vi "CRYView Model CurLibrary.vi"(8 "sOption":string, 9 "nData":i32, 10 "sData":string, 11 "sAction":string) -> (0 "bResult":bool=TRUE, 1 "pRefList_Out":variant[](array[variant]), 2 "pVIRef_Out":refnum<vi>, 3 "SData_Out":string)   [LabVIEW 2013]
uses:
  CRYNew View Global.vi
  CRYView Global.vi
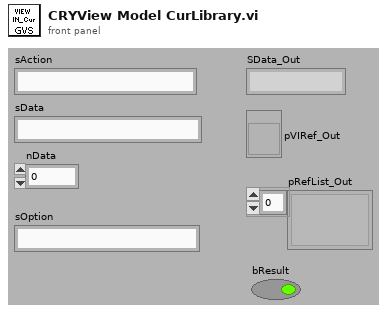
[diagram p1: front panel]
types:
  T1 = typedef "Graph Main Info Cluster.ctl" = cluster{"Selected_BarIdx":i32, "Selected_PanelIdx":i32, "Graph Main VIRef":refnum<vi>, "ToolBarClick":bool, "Spliter Ref Array":refnum<vi>[], "Panel Ref Array":refnum<vi>[], "Spliter_matrix":i32[][], "Panel_matrix":i32[][], "child_spliterIdx_matrix":i32[][], "split_pos_matrix":i32[][], "Title State":bool, "sQueueName":string, "Frame nID":i32, "Graph VIRef Array":cluster{"Graph VIRef":refnum<vi>, "Panel Idx":i32, "Frame VIRef":refnum<vi>, "Icon Ring":i32, "Graph Type":string}[], "View Type":string}
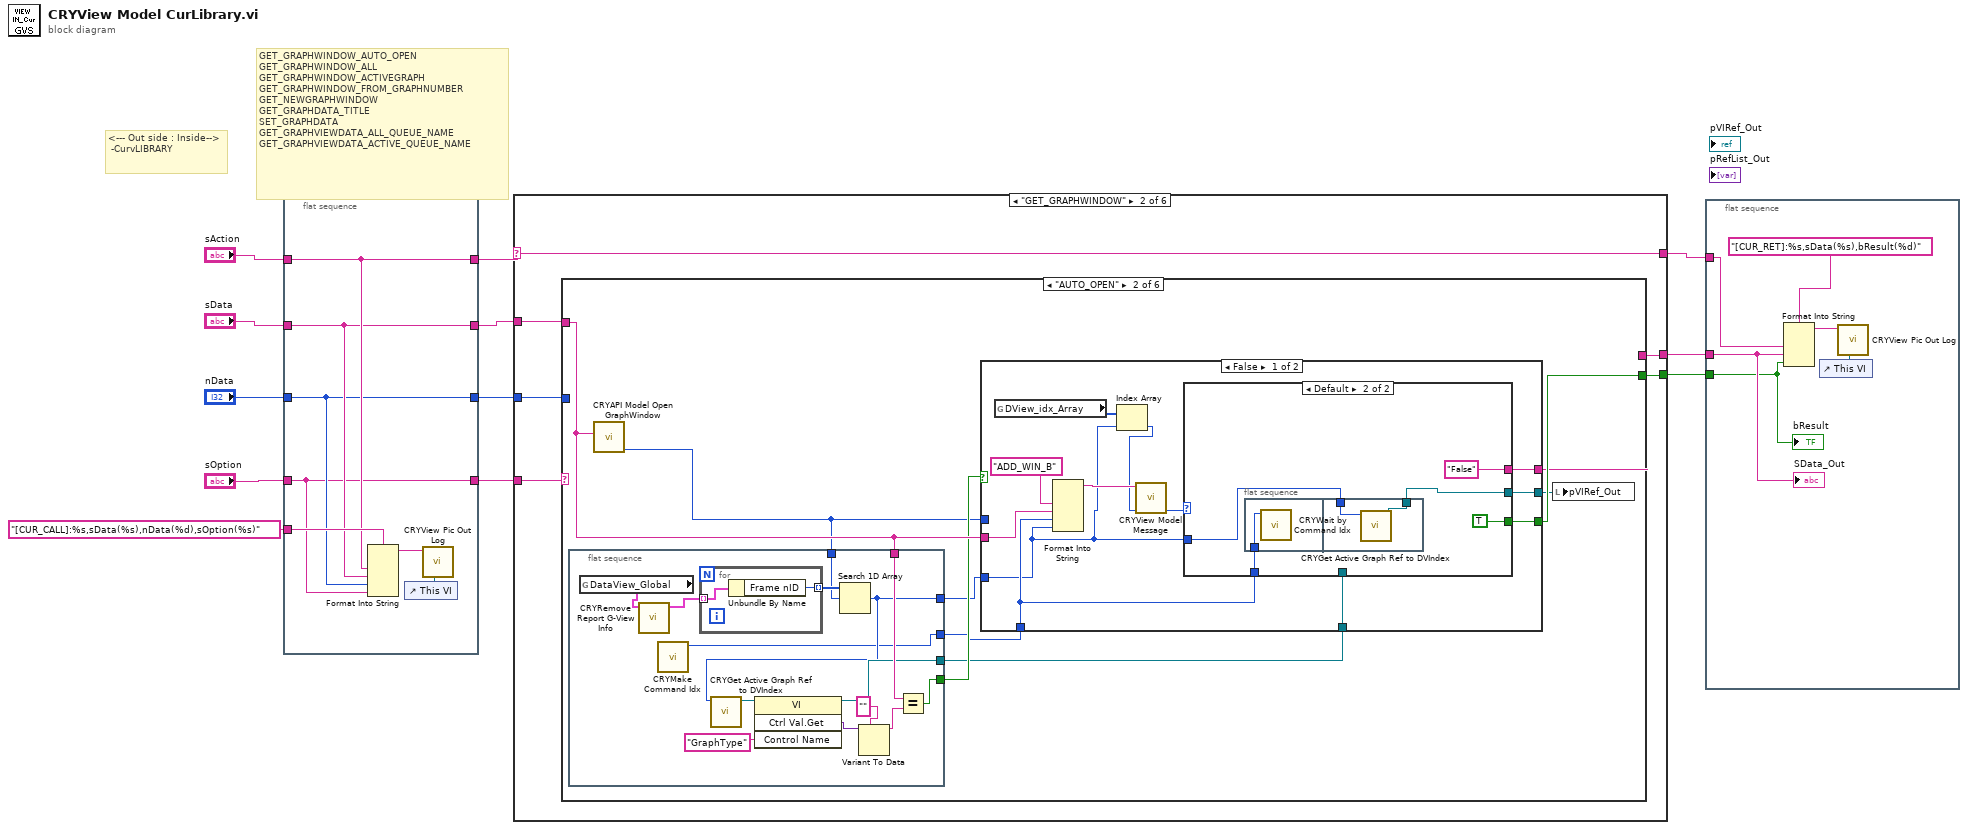
[diagram p0: block diagram]
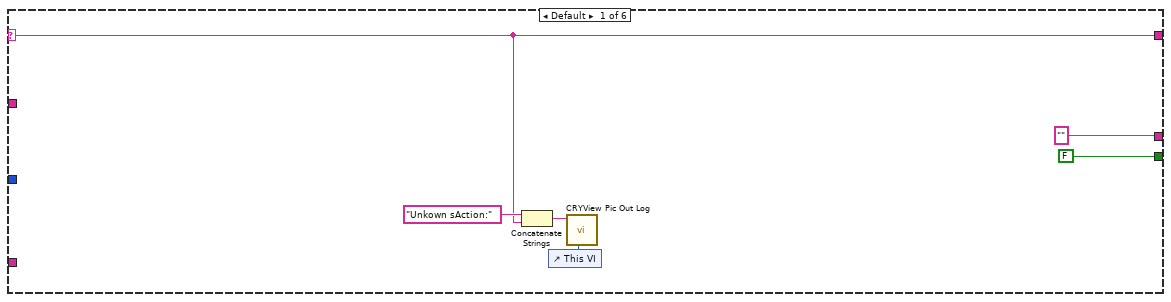
[diagram p2: hidden frame]
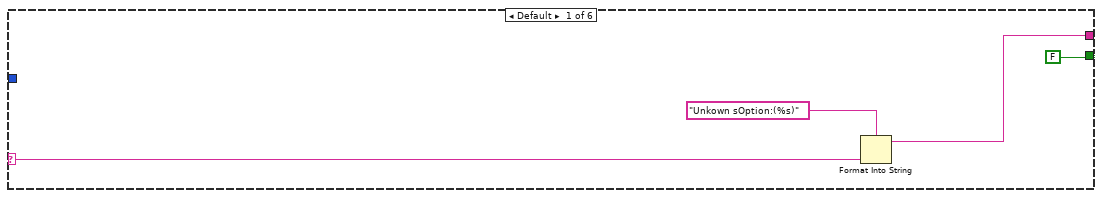
[diagram p3: hidden frame]
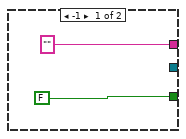
[diagram p4: hidden frame]
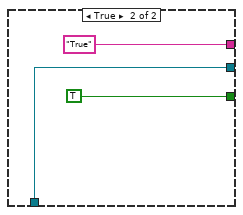
[diagram p5: hidden frame]
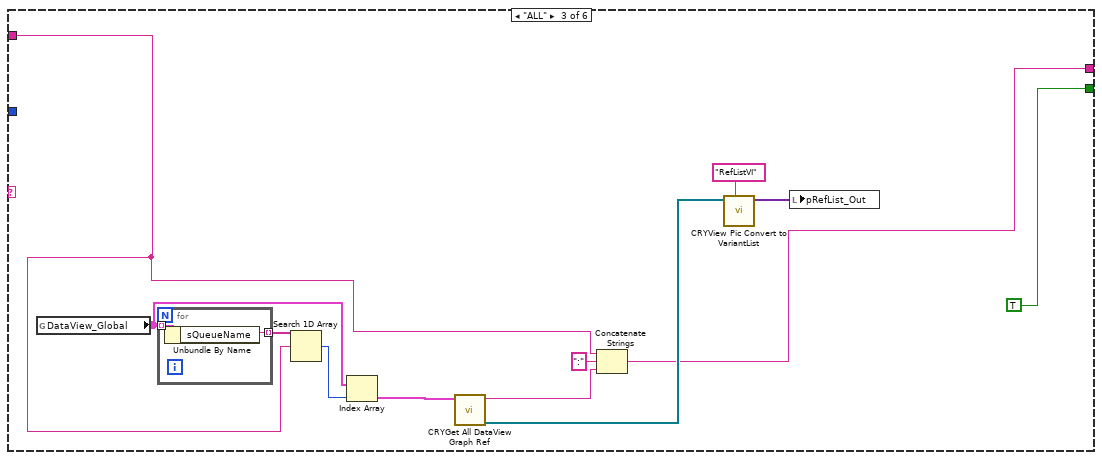
[diagram p6: hidden frame]
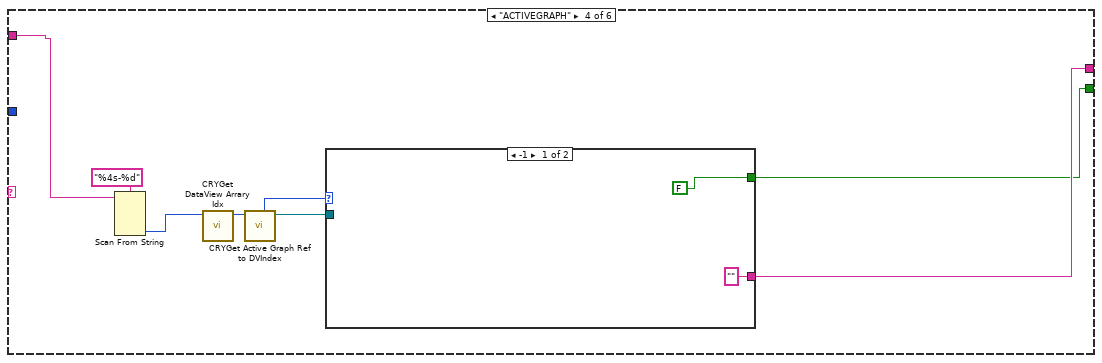
[diagram p7: hidden frame]
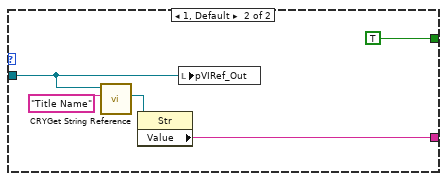
[diagram p8: hidden frame]
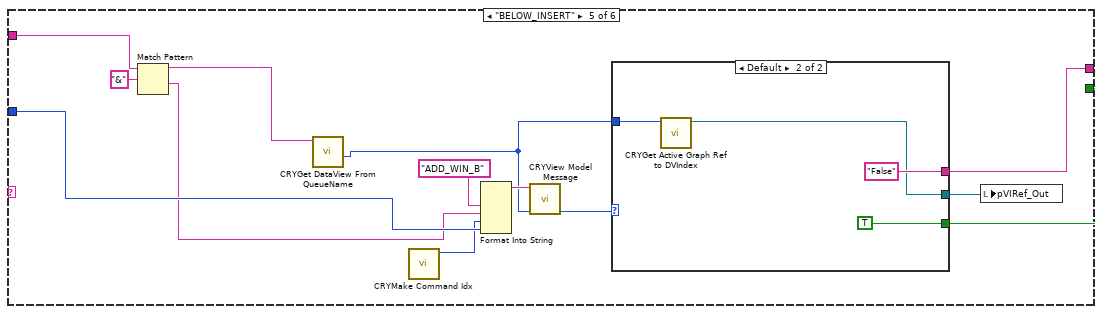
[diagram p9: hidden frame]
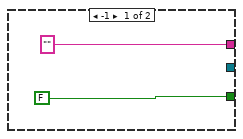
[diagram p10: hidden frame]
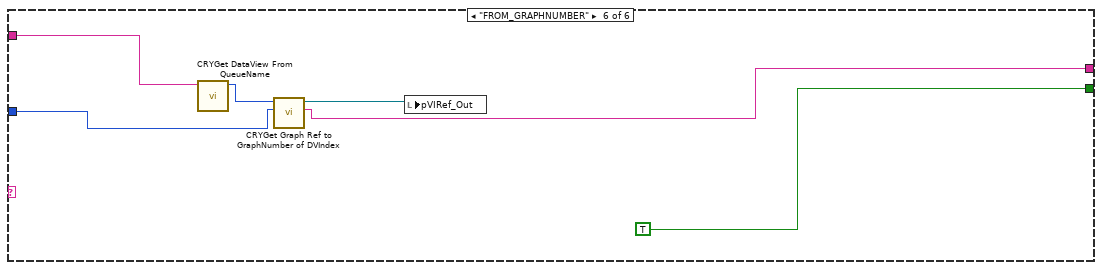
[diagram p11: hidden frame]
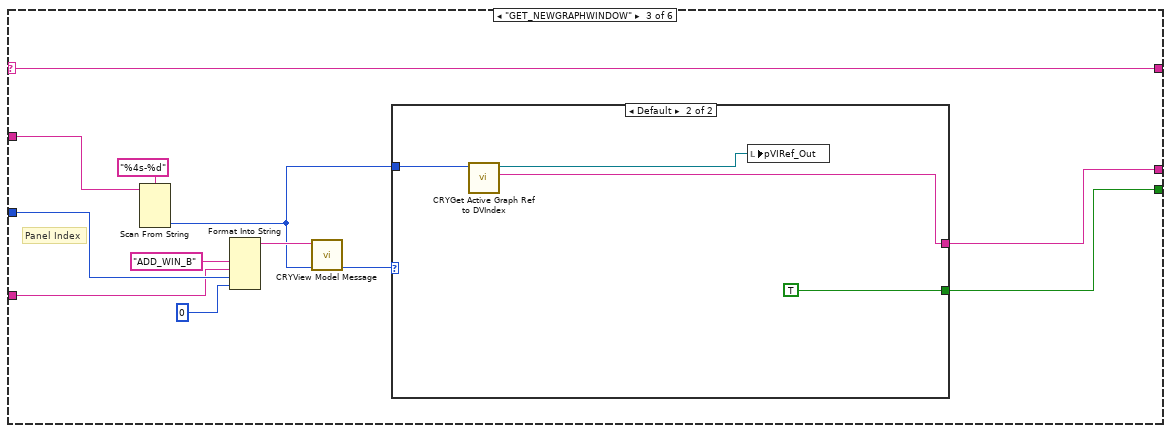
[diagram p12: hidden frame]
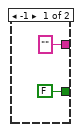
[diagram p13: hidden frame]
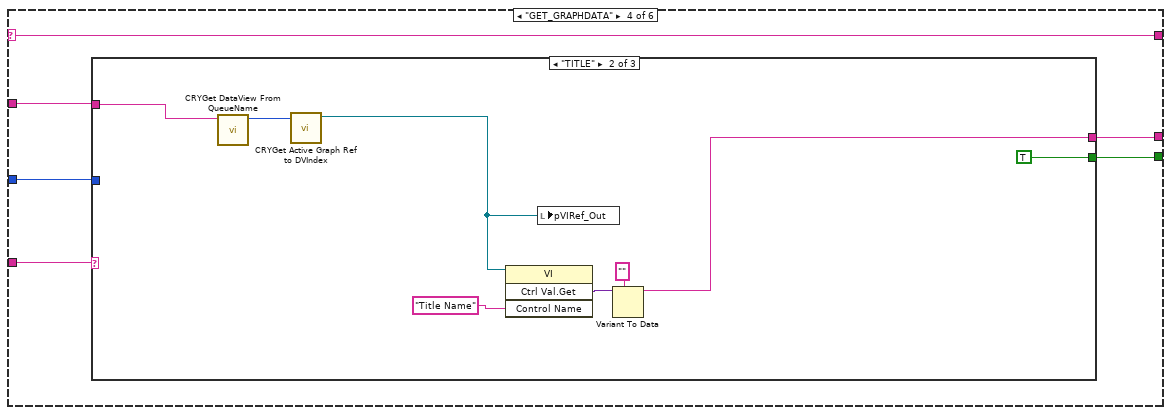
[diagram p14: hidden frame]
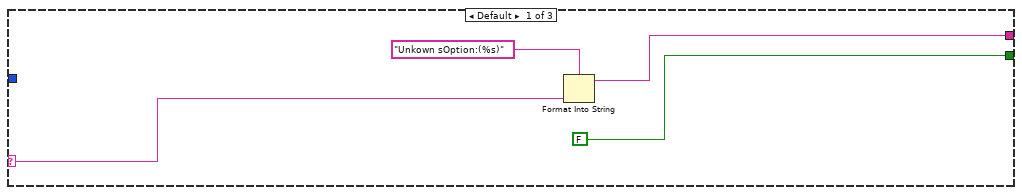
[diagram p15: hidden frame]
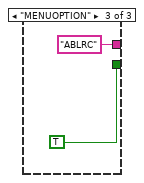
[diagram p16: hidden frame]
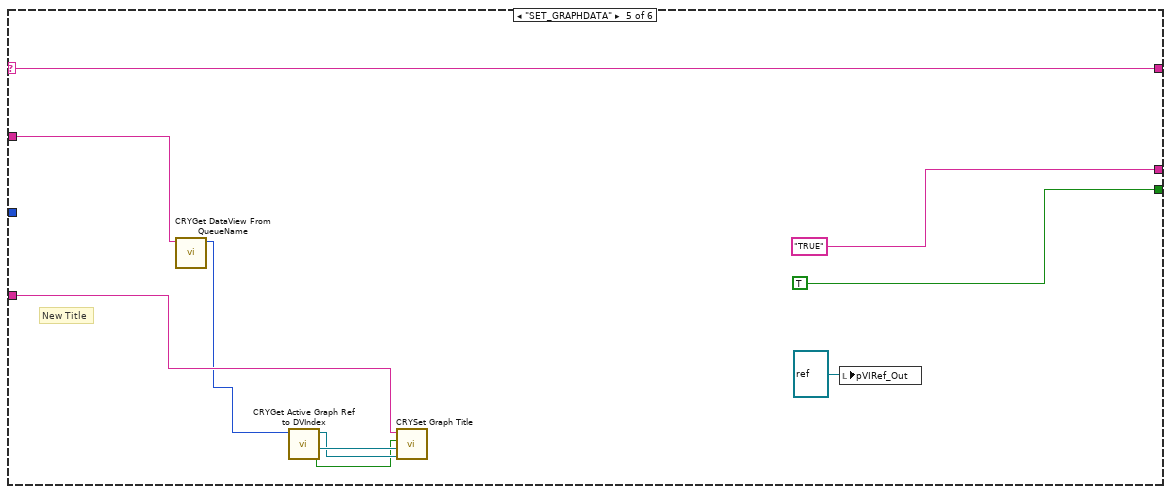
[diagram p17: hidden frame]
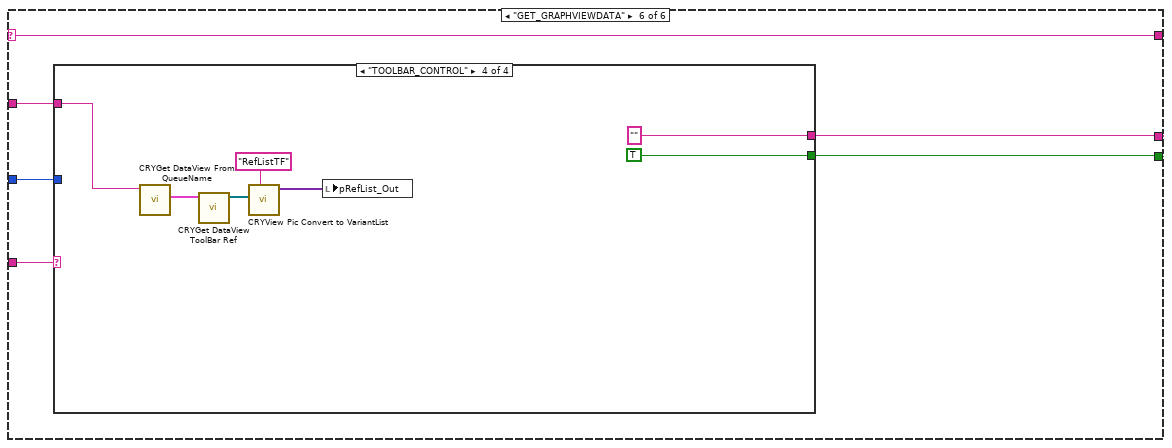
[diagram p18: hidden frame]
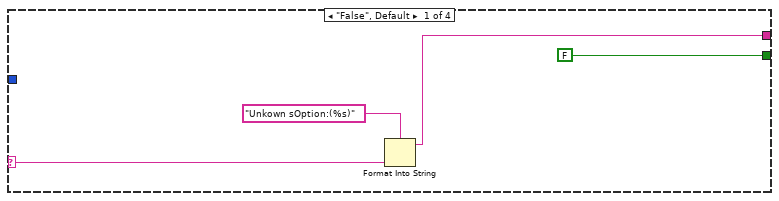
[diagram p19: hidden frame]
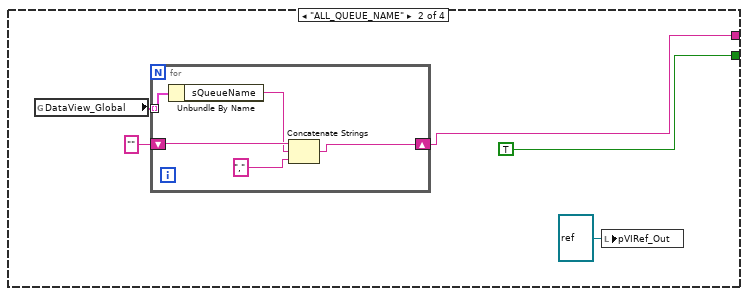
[diagram p20: hidden frame]
diagram:
  # "GET_GRAPHWINDOW_AUTO_OPEN\nGET_GRAPHWINDOW_ALL\nGET_GRAPHWINDOW_ACTIVEGRAPH\nGET_GRAPHWINDOW_FROM_GRAPHNUMBER\nGET_NEWGRAPHWINDOW\nGET_GRAPHDATA_TITLE\nSET_GRAPHDATA\nGET_GRAPHVIEWDATA_ALL_QUEUE_NAME\nGET_GRAPHVIEWDATA_ACTIVE_QUEUE_NAME"
  # "<--- Out side : Inside-->\n -CurvLIBRARY"
  n1 = flat-sequence {
    tunnel: [w16] -> w12
    tunnel: [w15] -> w11
    tunnel: [w14] -> w10
    tunnel: [w13] -> w9
    tunnel: "sData" -> [w15]
    tunnel: "nData" -> [w14]
    tunnel: "sOption" -> [w13]
    tunnel: "[CUR_CALL]:%s,sData(%s),nData(%d),sOption(%s)" ("format string") -> [w17]
    tunnel: "sAction" -> [w16]
    frame #0 {
      n2 = Format Into String(format string=w17, w16, w15, w14, w13) -> (resulting string=w18:string)  [unwired: 2 in, 1 out]
      n3 = control-ref of="This VI"() -> (w19:refnum<vi>)
      n4 = call "CRYView Pic Out Log.vi"("vi reference"=w19, "sData"=w18) -> ()  [unwired: 10 in]
    }
  }
  n5 = case shown="\"GET_GRAPHWINDOW\"" w12 {
    selector: w12 -> [w22 w31 w151 w163 w187 w193]
    tunnel: w9 -> [_ w26 w146 w158 w180 w190]
    tunnel: w11 -> [_ w28 w141 w160 w179 w189]
    tunnel: w10 -> [_ w27 w147 w159 _ w188]
    tunnel: [w22 w31 w151 w163 w187 w193] -> w7
    tunnel: ["" ("sAction") w30 w145 w162 "TRUE" ("Name") w192] -> w6
    tunnel: [FALSE w29 w144 w161 TRUE w191] -> w5
    frame Default {
      n6 = Concatenate Strings("Unkown sAction:" ("string"), w22) -> (w25:string)
      n7 = control-ref of="This VI"() -> (w23:refnum<vi>)
      n8 = call "CRYView Pic Out Log.vi"("vi reference"=w23, "sData"=w25) -> ()  [unwired: 10 in]
    }
    frame "GET_GRAPHWINDOW" {
      n9 = case shown="\"AUTO_OPEN\"" w26 {
        selector: w26 -> [w33 _ _ _ _ _]
        tunnel: [w32 w43 w86 w102 w123 w136] -> w30
        tunnel: [FALSE w44 TRUE w100 w122 TRUE] -> w29
        tunnel: w28 -> [_ w41 w88 w103 w120 w134]
        tunnel: w27 -> [_ _ _ _ w121 w138]
        frame Default {
          n10 = Format Into String(format string="Unkown sOption:(%s)", w33) -> (resulting string=w32:string)  [unwired: 2 in, 1 out]
        }
        frame "AUTO_OPEN" {
          n11 = flat-sequence {
            tunnel: w41 -> [w58]
            tunnel: [w57] -> w40
            tunnel: [w53] -> w39
            tunnel: w38 -> [w49]
            tunnel: [w48] -> w37
            tunnel: [w47] -> w36
            frame #0 {
              n12 = global read "CRYNew View Global.vi" "DataView_Global"() -> (w46:T1[])
              n13 = call "CRYRemove Report G-View Info.vi"("DataView_Info Array"=w46) -> ("DataView_Info Array out"=w45:T1[])  [unwired: 9 in, 1 out]
              n14 = call "CRYMake Command Idx.vi"() -> ("New Command Idx"=w47:i32)  [unwired: 11 in]
              n15 = for {
                tunnel: [w60] -> w50 mode=indexing
                tunnel: w45 -> [w59] mode=indexing
                n16 = Unbundle By Name(w59) -> ("Frame nID"=w60:i32)
              }
              n17 = Search 1D Array(1D array=w50, element=w49) -> (index of element=w48:i32)  [unwired: 1 in]
              n18 = call "CRYGet Active Graph Ref to DVIndex.vi"("DV Array index"=w48) -> ("Inserted Graph VIRef out"=w56:refnum<vi>)  [unwired: 5 in, 5 out]
              n19 = invoke class="VI" method="Ctrl Val.Get"(reference=w56, "Control Name"="GraphType") -> (reference out=w53:refnum<vi>, "Get Control Value Variant"=w54:variant)  [unwired: 2 in, 2 out]
              n20 = Variant To Data(type="" ("Control Name"), Variant=w54) -> (data=w51:string)  [unwired: 1 in, 1 out]
              n21 = Equal?(x=w58, y=w51) -> (x = y?=w57:bool)
            }
          }
          n22 = call "CRYAPI Model Open GraphWindow.vi"("sData"=w41) -> ("nID"=w38:i32)  [unwired: 9 in, 1 out]
          n23 = case shown="False" w40 {
            tunnel: w41 -> [w71 _]
            tunnel: w38 -> [_ _]
            tunnel: [w69 TRUE ("bResult")] -> w44
            tunnel: [w68 w83] -> w42
            tunnel: [w67 "True" ("sIcon")] -> w43
            tunnel: w39 -> [w65 w83]
            tunnel: w37 -> [w62 _]
            tunnel: w36 -> [w64 _]
            frame False {
              n24 = global read "CRYNew View Global.vi" "DView_idx_Array"() -> (w63:i32[])
              n25 = Format Into String("ADD_WIN_B" ("input 1"), w71, w64, w62) -> (resulting string=w70:string)  [unwired: 3 in, 1 out]
              n26 = Index Array(array=w63, index=w62) -> (element=w61:i32)
              n27 = call "CRYView Model Message.vi"("nData"=w61, "sMsgData"=w70) -> ("nData_Out"=w66:i32)  [unwired: 7 in, 2 out]
              n28 = case shown="Default" w66 {
                tunnel: [_ w75] -> w68
                tunnel: [FALSE ("bResult") TRUE ("bResult")] -> w69
                tunnel: ["" ("sIcon") "False" ("sIcon")] -> w67
                tunnel: w65 -> [_ _]
                tunnel: w62 -> [_ w76]
                tunnel: w64 -> [_ w77]
                frame -1 {
                }
                frame Default {
                  n29 = flat-sequence {
                    tunnel: w77 -> [w80]
                    tunnel: w76 -> [w82]
                    tunnel: [w81] -> w75
                    frame #0 {
                      n30 = call "CRYWait by Command Idx.vi"("New Command Idx"=w80) -> ()  [unwired: 11 in]
                    }
                    frame #1 {
                      n31 = call "CRYGet Active Graph Ref to DVIndex.vi"("DV Array index"=w82) -> ("Inserted Graph VIRef out"=w81:refnum<vi>)  [unwired: 5 in, 5 out]
                    }
                  }
                }
              }
            }
            frame True {
            }
          }
          n32 = local write "pVIRef_Out"(w42) -> ()
        }
        frame "ALL" {
          n33 = global read "CRYNew View Global.vi" "DataView_Global"() -> (w92:T1[])
          n34 = for {
            tunnel: w92 -> [w99] mode=indexing
            tunnel: [w98] -> w94 mode=indexing
            n35 = Unbundle By Name(w99) -> ("sQueueName"=w98:string)
          }
          n36 = Search 1D Array(1D array=w94, element=w88) -> (index of element=w93:i32)  [unwired: 1 in]
          n37 = Index Array(array=w92, index=w93) -> (element=w91:T1)
          n38 = call "CRYGet All DataView Graph Ref.vi"("DataViewb in"=w91) -> ("Graph VIRef Out"=w90:refnum<vi>[], "sName Array Out"=w87:string)  [unwired: 9 in]
          n39 = Concatenate Strings(w88, ":" ("string"), w87) -> (w86:string)
          n40 = call "CRYView Pic Convert to VariantList.vi"("sAction"="RefListVI", "pRefListVI"=w90) -> ("RefList_Out"=w95:variant[])  [unwired: 9 in]
          n41 = local write "pRefList_Out"(w95) -> ()
        }
        frame "ACTIVEGRAPH" {
          n42 = Scan From String(format string="%4s-%d", input string=w103) -> (output 2=w106:i32)  [unwired: 5 in, 3 out]
          n43 = call "CRYGet DataView Arrary Idx.vi"("DataView Idx In"=w106) -> ("DataView Arrary Idx out"=w105:i32)  [unwired: 10 in]
          n44 = call "CRYGet Active Graph Ref to DVIndex.vi"("DV Array index"=w105) -> ("Inserted Graph VIRef out"=w104:refnum<vi>, "Graph VIRef Array Index"=w101:i32)  [unwired: 5 in, 4 out]
          n45 = case shown="-1" w101 {
            tunnel: w104 -> [_ w112]
            tunnel: ["" ("Value") w111] -> w102
            tunnel: [FALSE ("bResult") TRUE ("bResult")] -> w100
            frame -1 {
            }
            frame 1, Default {
              n46 = call "CRYGet String Reference.vi"("Label Name"="Title Name", "VI Refnum"=w112) -> ("String Ref Out"=w113:refnum<vi>)  [unwired: 7 in, 2 out]
              n47 = property class="Str"(reference=w113) -> ("Value"=w111:string)  [unwired: 1 in, 2 out]
              n48 = local write "pVIRef_Out"(w112) -> ()
            }
          }
        }
        frame "BELOW_INSERT" {
          n49 = Match Pattern(string=w120, regular expression="&") -> (before substring=w117:string, after substring=w118:string)  [unwired: 1 in, 2 out]
          n50 = call "CRYGet DataView From QueueName.vi"("DataView QueueName"=w117) -> ("DataView Idx out"=w116:i32)  [unwired: 8 in, 2 out]
          n51 = call "CRYMake Command Idx.vi"() -> ("New Command Idx"=w115:i32)  [unwired: 11 in]
          n52 = Format Into String("ADD_WIN_B" ("input 1"), w118, w115, w121) -> (resulting string=w126:string)  [unwired: 3 in, 1 out]
          n53 = call "CRYView Model Message.vi"("nData"=w116, "sMsgData"=w126) -> ("nData_Out"=w125:i32)  [unwired: 7 in, 2 out]
          n54 = case shown="Default" w125 {
            tunnel: [_ w131] -> w124
            tunnel: [FALSE ("bResult") TRUE ("bResult")] -> w122
            tunnel: ["" ("sIcon") "False" ("sIcon")] -> w123
            tunnel: w116 -> [_ w130]
            frame -1 {
            }
            frame Default {
              n55 = call "CRYGet Active Graph Ref to DVIndex.vi"("DV Array index"=w130) -> ("Inserted Graph VIRef out"=w131:refnum<vi>)  [unwired: 5 in, 5 out]
            }
          }
          n56 = local write "pVIRef_Out"(w124) -> ()
        }
        frame "FROM_GRAPHNUMBER" {
          n57 = call "CRYGet DataView From QueueName.vi"("DataView QueueName"=w134) -> ("DataView Arrary Idx out"=w135:i32)  [unwired: 8 in, 2 out]
          n58 = call "CRYGet Graph Ref to GraphNumber of DVIndex.vi"("Graph Number"=w138, "DV Array index"=w135) -> ("sQueueName"=w136:string, "Inserted Graph VIRef out"=w137:refnum<vi>)  [unwired: 7 in, 1 out]
          n59 = local write "pVIRef_Out"(w137) -> ()
        }
      }
    }
    frame "GET_NEWGRAPHWINDOW" {
      # "Panel Index"
      n60 = Scan From String(format string="%4s-%d", input string=w141) -> (output 2=w140:i32)  [unwired: 5 in, 3 out]
      n61 = Format Into String("ADD_WIN_B" ("input 1"), w146, w147, 0 ("input 4")) -> (resulting string=w149:string)  [unwired: 3 in, 1 out]
      n62 = call "CRYView Model Message.vi"("nData"=w140, "sMsgData"=w149) -> ("nData_Out"=w143:i32)  [unwired: 7 in, 2 out]
      n63 = case shown="Default" w143 {
        tunnel: ["" ("sName") w154] -> w145
        tunnel: [FALSE TRUE] -> w144
        tunnel: w140 -> [_ w156]
        frame -1 {
        }
        frame Default {
          n64 = call "CRYGet Active Graph Ref to DVIndex.vi"("DV Array index"=w156) -> ("sQueueName"=w154:string, "Inserted Graph VIRef out"=w155:refnum<vi>)  [unwired: 5 in, 4 out]
          n65 = local write "pVIRef_Out"(w155) -> ()
        }
      }
    }
    frame "GET_GRAPHDATA" {
      n66 = case shown="\"TITLE\"" w158 {
        selector: w158 -> [w166 _ _]
        tunnel: w160 -> [_ w174 _]
        tunnel: w159 -> [_ _ _]
        tunnel: [w165 w169 "ABLRC"] -> w162
        tunnel: [FALSE TRUE TRUE] -> w161
        frame Default {
          n67 = Format Into String(format string="Unkown sOption:(%s)", w166) -> (resulting string=w165:string)  [unwired: 2 in, 1 out]
        }
        frame "TITLE" {
          n68 = call "CRYGet DataView From QueueName.vi"("DataView QueueName"=w174) -> ("DataView Arrary Idx out"=w173:i32)  [unwired: 8 in, 2 out]
          n69 = call "CRYGet Active Graph Ref to DVIndex.vi"("DV Array index"=w173) -> ("Inserted Graph VIRef out"=w171:refnum<vi>)  [unwired: 5 in, 5 out]
          n70 = invoke class="VI" method="Ctrl Val.Get"(reference=w171, "Control Name"="Title Name" ("Label Name")) -> ("Get Control Value Variant"=w170:variant)  [unwired: 2 in, 3 out]
          n71 = local write "pVIRef_Out"(w171) -> ()
          n72 = Variant To Data(type="" ("Label Name"), Variant=w170) -> (data=w169:string)  [unwired: 1 in, 1 out]
        }
        frame "MENUOPTION" {
        }
      }
    }
    frame "SET_GRAPHDATA" {
      # "New Title"
      n73 = call "CRYGet DataView From QueueName.vi"("DataView QueueName"=w179) -> ("DataView Arrary Idx out"=w178:i32)  [unwired: 8 in, 2 out]
      n74 = call "CRYGet Active Graph Ref to DVIndex.vi"("DV Array index"=w178) -> ("Title State"=w181:bool, "Frame VIRef"=w183:refnum<vi>, "Inserted Graph VIRef out"=w182:refnum<vi>)  [unwired: 5 in, 3 out]
      n75 = call "CRYSet Graph Title.vi"("Inserted Graph VIRef out"=w182, "Frame VIRef"=w183, "Title State"=w181, "Title Name in"=w180) -> ()  [unwired: 7 in, 1 out]
      n76 = local write "pVIRef_Out"(refnum<vi> refnum ("pVIRef_Out")) -> ()
    }
    frame "GET_GRAPHVIEWDATA" {
      n77 = case shown="\"TOOLBAR_CONTROL\"" w190 {
        selector: w190 -> [w194 _ _ _]
        tunnel: [w196 w200 w212 "" ("sName")] -> w192
        tunnel: [FALSE TRUE w211 TRUE] -> w191
        tunnel: w189 -> [_ _ _ w227]
        tunnel: w188 -> [_ _ _ _]
        frame "False", Default {
          n78 = Format Into String(format string="Unkown sOption:(%s)", w194) -> (resulting string=w196:string)  [unwired: 2 in, 1 out]
        }
        frame "ALL_QUEUE_NAME" {
          n79 = global read "CRYNew View Global.vi" "DataView_Global"() -> (w198:T1[])
          n80 = for {
            tunnel: w198 -> [w207] mode=indexing
            shift-right: [w205] -> w200
            shift-left: "" -> [w206]
            n81 = Unbundle By Name(w207) -> ("sQueueName"=w203:string)
            n82 = Concatenate Strings(w206, w203, ",") -> (w205:string)
          }
          n83 = local write "pVIRef_Out"(refnum<vi> refnum ("pVIRef_Out")) -> ()
        }
        frame "ACTIVE_QUEUE_NAME" {
          n84 = call "CRYEqual DataView Idx and Actived Wnd.vi"() -> ("DataView QueueName"=w208:string, "DataView Index"=w209:i32)  [unwired: 9 in, 1 out]
          n85 = case shown="-1" w209 {
            tunnel: [w214 TRUE] -> w211
            tunnel: [w215 w223] -> w212
            tunnel: w208 -> [_ w223]
            frame -1 {
              n86 = global read "CRYView Global.vi" "sActiveView"() -> (w217:string)
              n87 = call "CRYGet DataView From QueueName Except Report.vi"("DataView QueueName"=w217) -> ("DataView out"=w213:T1, "DataView Arrary Idx out"=w216:i32)  [unwired: 8 in, 1 out]
              n88 = case shown="0, Default" w216 {
                tunnel: [w220 ""] -> w215
                tunnel: [TRUE FALSE] -> w214
                tunnel: w213 -> [w218 _]
                frame 0, Default {
                  n89 = Unbundle By Name(w218) -> ("sQueueName"=w220:string)
                }
                frame -1 {
                }
              }
            }
            frame 0, Default {
            }
          }
          n90 = local write "pVIRef_Out"(refnum<vi> refnum ("pVIRef_Out")) -> ()
        }
        frame "TOOLBAR_CONTROL" {
          n91 = call "CRYGet DataView From QueueName.vi"("DataView QueueName"=w227) -> ("DataView out"=w226:T1)  [unwired: 8 in, 2 out]
          n92 = call "CRYGet DataView ToolBar Ref.vi"("DataViewb in"=w226) -> ("pRefListTF_Out"=w225:refnum<vi>[])  [unwired: 10 in]
          n93 = call "CRYView Pic Convert to VariantList.vi"("sAction"="RefListTF", "pRefListTF"=w225) -> ("RefList_Out"=w230:variant[])  [unwired: 9 in]
          n94 = local write "pRefList_Out"(w230) -> ()
        }
      }
    }
  }
  n95 = flat-sequence {
    tunnel: w5 -> [w232]
    tunnel: w6 -> [w233]
    tunnel: w7 -> [w234]
    frame #0 {
      n96 = Format Into String(format string="[CUR_RET]:%s,sData(%s),bResult(%d)", w234, w233, w232) -> (resulting string=w236:string)  [unwired: 2 in, 1 out]
      n97 = control-ref of="This VI"() -> (w237:refnum<vi>)
      n98 = call "CRYView Pic Out Log.vi"("vi reference"=w237, "sData"=w236) -> ()  [unwired: 10 in]
      "SData_Out" <- w233
      "bResult" <- w232
    }
  }
